vi "Get Primary Destination Path.vi"(8 "error in (no error)":errorcluster, 11 "NI_AB_API_Build in":refnum<class "NI_AB_API_Build.lvclass">) -> (0 "error out":errorcluster, 2 "Primary destination path":path, 3 "NI_AB_API_Build out":refnum<class "NI_AB_API_Build.lvclass">)   [LabVIEW 2020, in "NI_AB_API_Build.lvclass"]
uses:
  <vilib>/AppBuilder/AB_API/Build/NI_AB_API_Build.lvclass
  <vilib>/AppBuilder/AB_API/Build/NI_AB_API_Build.lvclass/NI_AB_API_Build.ctl
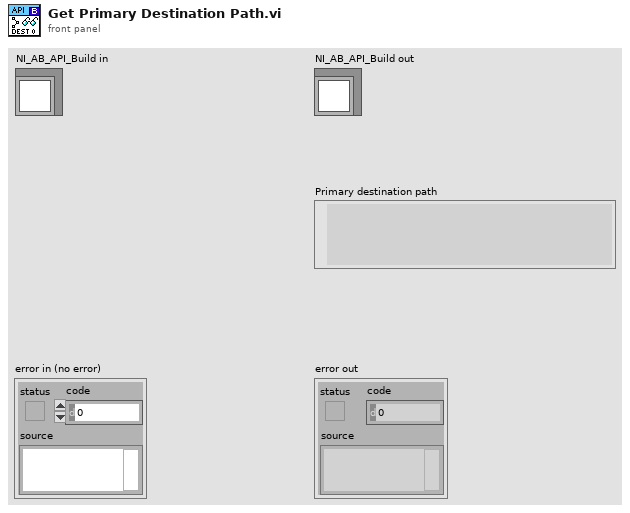
[diagram p1: front panel]
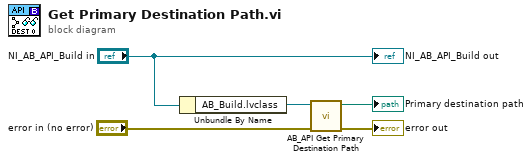
[diagram p0: block diagram]
diagram:
  n1 = Unbundle By Name("NI_AB_API_Build in") -> ("AB_Build.lvclass"=w1:refnum<class "AB_Build.lvclass">)
  n2 = call <vilib>:"AB_API Get Primary Destination Path.vi"("error in (no error)"="error in (no error)", "Build in"=w1) -> ("error out"=→"error out":errorcluster, "primary destination path"=→"Primary destination path":path)  [unwired: 8 out]
  "NI_AB_API_Build out" <- "NI_AB_API_Build in"
